vi "Main UI.vi"() -> ()   [LabVIEW 2013]
uses:
  SubVi/Global constant.vi
  <vilib>/regexp/Match Regular Expression.xnode
panel:
  out "Name":string
  out "Info":cluster{"PASS":u32, "Total":u32, "Rate %":dbl}
  out "Test Time (s)":string
  out "MainProcess":T1(ring)
  out "SN":string
  in  "Cancel Button":bool
  out "Model":string
  out "Result":string
  in  "OK Button":bool
  in  "Multicolumn Listbox":i32(listbox)
  out "Horizontal Graduated Bar":u8(slide) max=28 scale=-1.0..8.0
  out "reslut":bool
  out "Boolean":bool
  out "?":string[](array[string])
  out "ItemTag":string
  # "Powered by Domi"
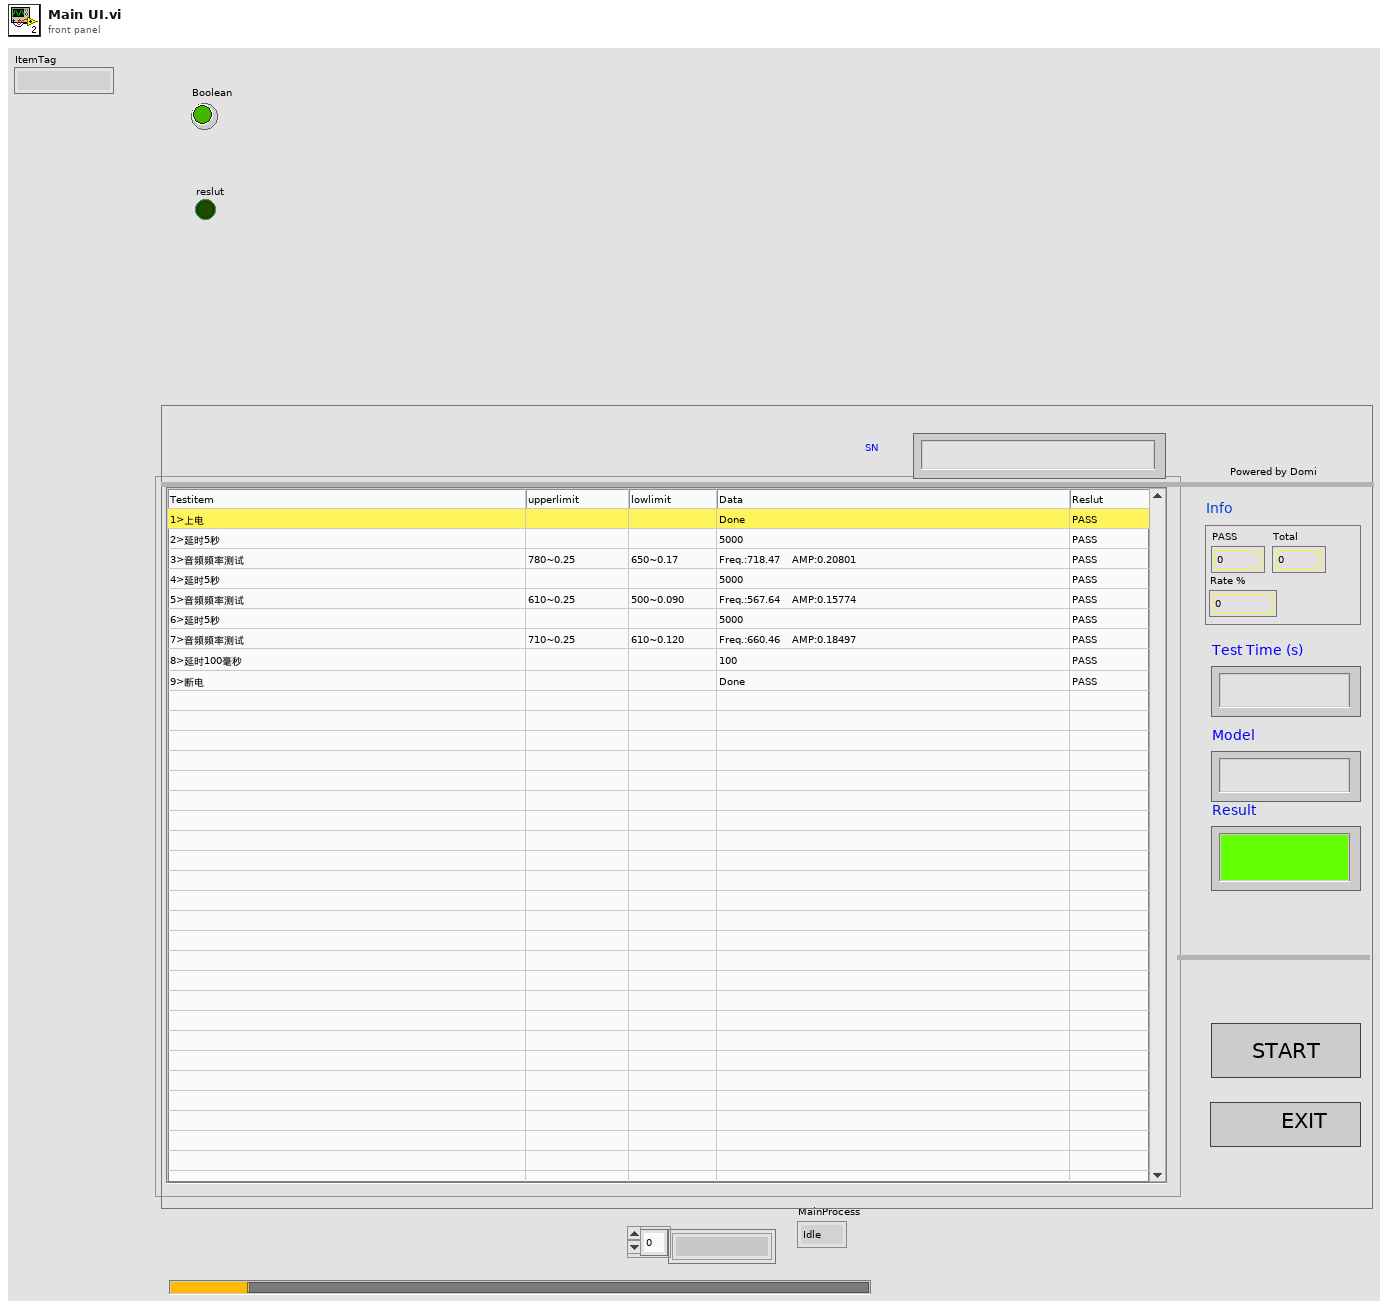
[diagram p1: front panel]
types:
  T1 = enum16{"Idle", "SystemInit", "SpecialEvent", "Barcode(SN)", "TestInitialize", "Test", "TestEnd", "SaveTestData", "Exit", "Stop"}
  T2 = enum8{"Enabled", "Disabled", "Disabled and Grayed Out"}
  T3 = enum16{"open", "replace", "create", "open or create", "replace or create", "replace or create with confirmation"}
  T4 = cluster{"step name 1":string, "updata 2":string, "limitdata 3":string, "load vi name 4":string, "parameter 5":string}
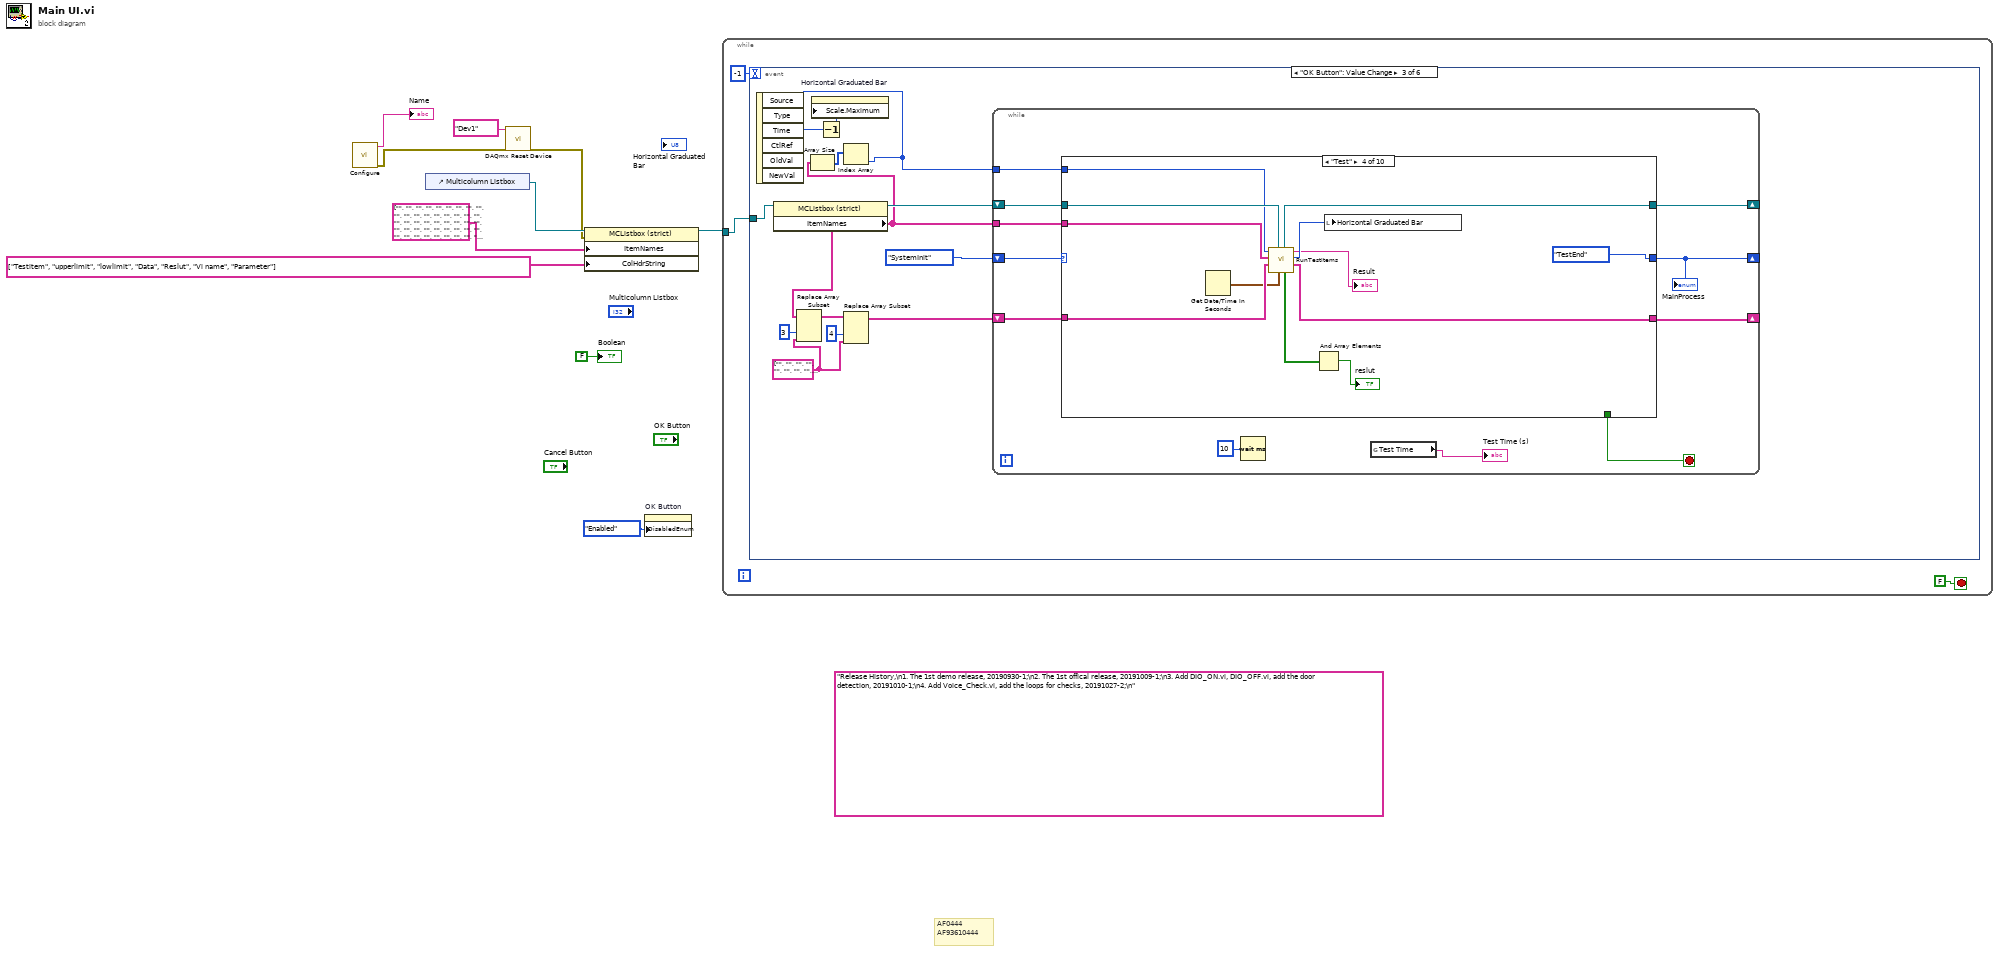
[diagram p0: block diagram]
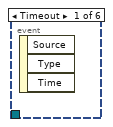
[diagram p2: hidden frame]
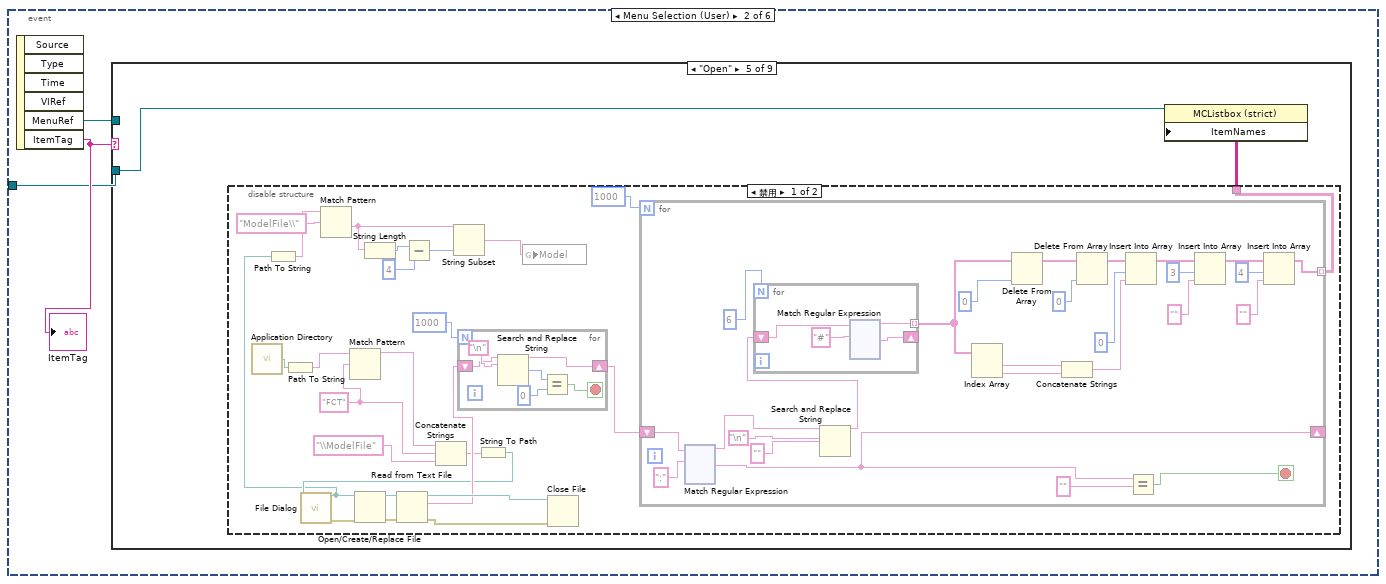
[diagram p3: hidden frame]
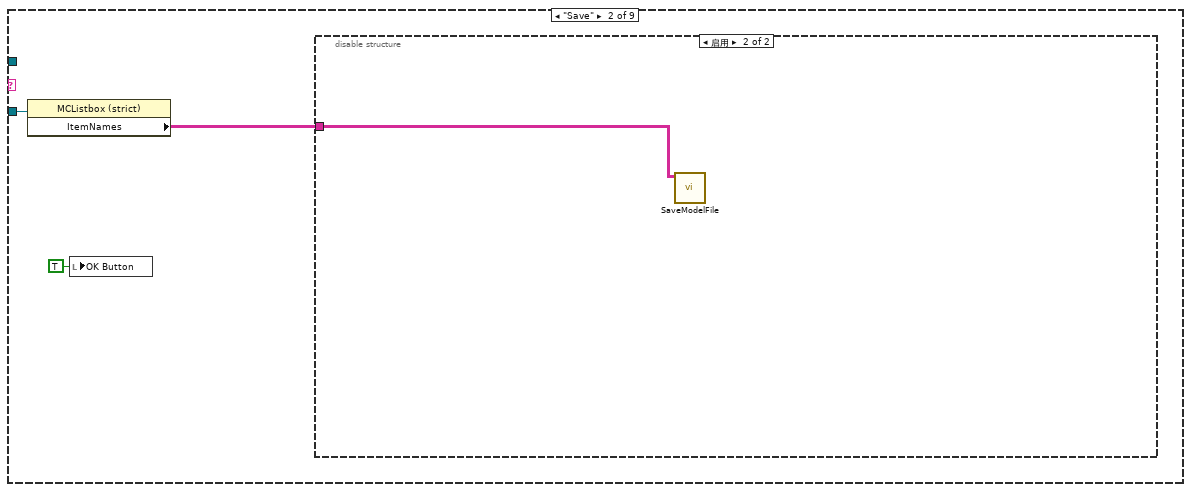
[diagram p5: hidden frame]
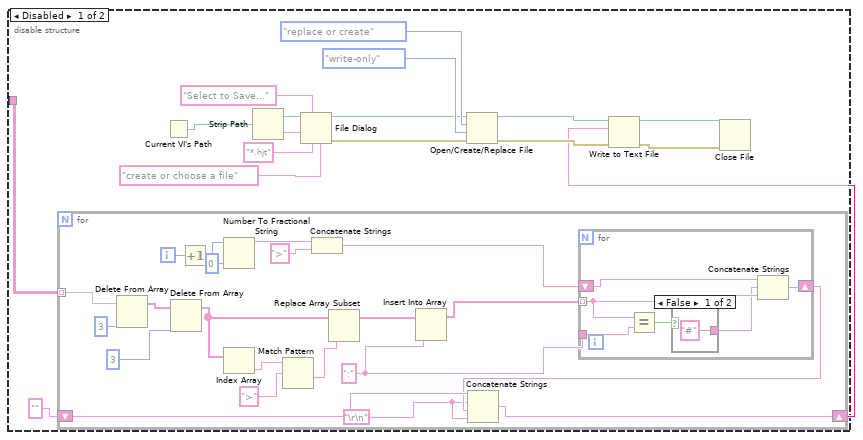
[diagram p6: hidden frame]
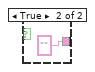
[diagram p7: hidden frame]
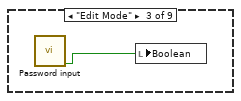
[diagram p8: hidden frame]
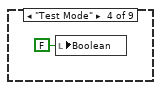
[diagram p9: hidden frame]
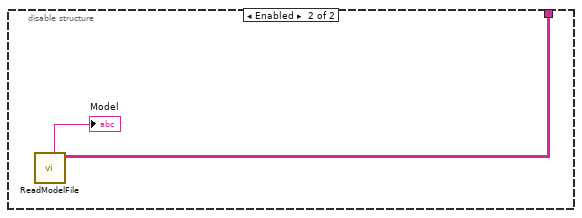
[diagram p10: hidden frame]
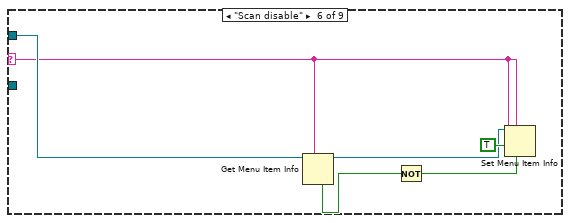
[diagram p11: hidden frame]
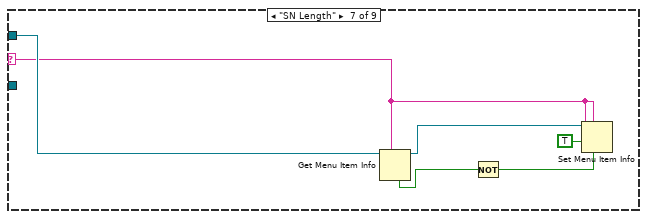
[diagram p12: hidden frame]
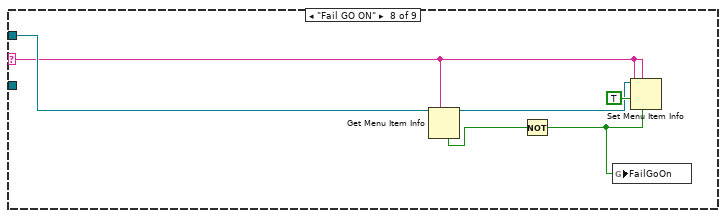
[diagram p13: hidden frame]
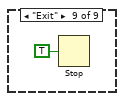
[diagram p14: hidden frame]
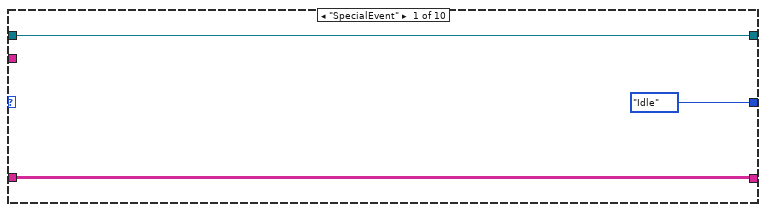
[diagram p15: hidden frame]
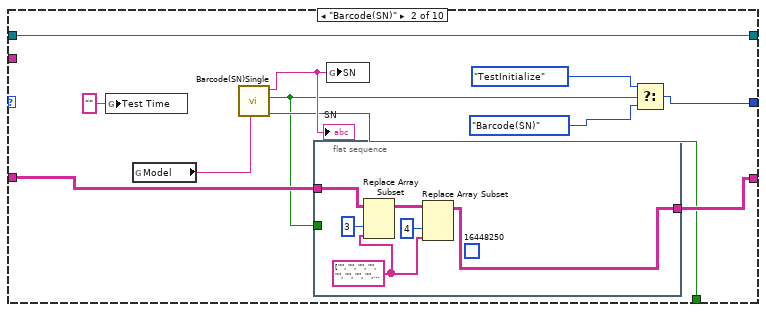
[diagram p16: hidden frame]
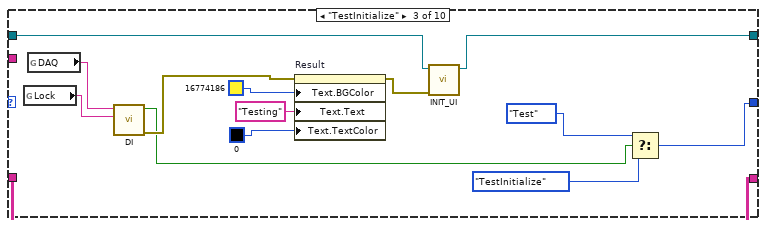
[diagram p17: hidden frame]
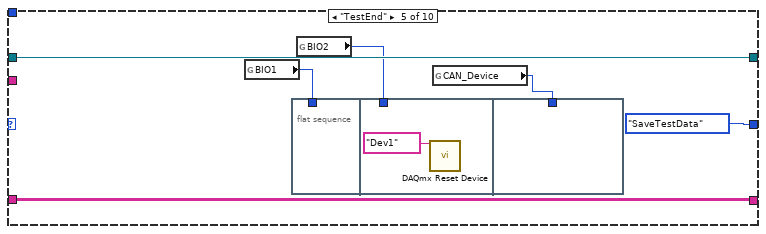
[diagram p18: hidden frame]
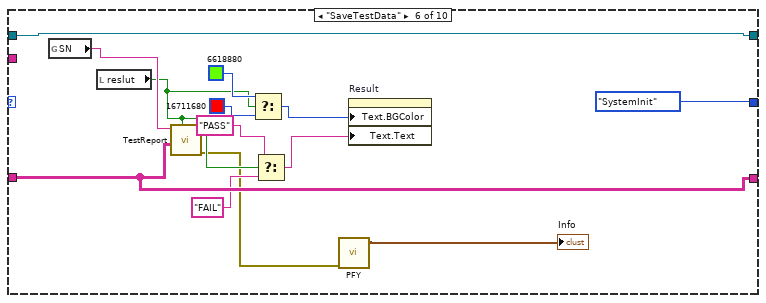
[diagram p19: hidden frame]
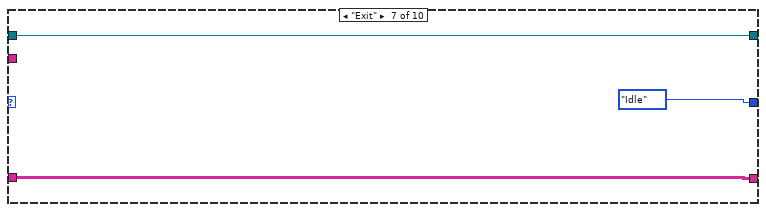
[diagram p20: hidden frame]
diagram:
  (unwired) "Release History,\n1. The 1st demo release, 20190930-1;\n2. The 1st offical release, 20191009-1;\n3. Add DIO_ON.vi, DIO_OFF.vi, add the door detection, 20191010-1;\n4. Add Voice_Check.vi, add the loops for checks, 20191027-2;\n"
  # "AF0444\nAF93610444"
  n1 = call "Configure.vi"() -> ("error out"=w2:errorcluster, "name"=→"Name":string)  [unwired: 10 in]
  n2 = control-ref of="Multicolumn Listbox"() -> (w10:refnum<vi>)
  n3 = call <vilib>:"DAQmx Reset Device.vi"("device in"=tag "Dev1", "error in"=w2) -> ("error out"=w3:errorcluster)  [unwired: 13 in]
  n4 = property class="MCListbox (strict)"(reference=w10, error in=w3, "ItemNames"=string[][] [["", "", "", "", "", "", "", ""], ["", "", "", "", "", "", "", ""], ["", "", "", "", "", "", "", ""], ["", "", "", "", "", "", "", ""], ["", "", "", "", "", "", "", ""], ["", "", "", "", "", "", "", ""], ["", "", "", "", "", "", "", ""], ["", "", "", "", "", "", "", ""], ["", "", "", "", "", "", "", ""], ["", "", "", "", "", "", "", ""], ["", "", "", "", "", "", "", ""], ["", "", "", "", "", "", "", ""], ["", "", "", "", "", "", "", ""], ["", "", "", "", "", "", "", ""], ["", "", "", "", "", "", "", ""], ["", "", "", "", "", "", "", ""], ["", "", "", "", "", "", "", ""], ["", "", "", "", "", "", "", ""], ["", "", "", "", "", "", "", ""], ["", "", "", "", "", "", "", ""], ["", "", "", "", "", "", "", ""], ["", "", "", "", "", "", "", " "], ["", "", "", "", "", "", "", ""], ["", "", "", "", "", "", "", ""], ["", "", "", "", "", "", "", ""], ["", "", "", "", "", "", "", ""], ["", "", "", "", "", "", "", ""], ["", "", "", "", "", "", "", ""], ["", "", "", "", "", "", "", ""], ["", "", "", "", "", "", "", ""], ["", "", "", "", "", "", "", ""], ["", "", "", "", "", "", "", ""], ["", "", "", "", "", "", "", ""], ["", "", "", "", "", "", "", ""], ["", "", "", "", "", "", "", ""], ["", "", "", "", "", "", "", ""], ["", "", "", "", "", "", "", ""], ["", "", "", "", "", "", "", ""], ["", "", "", "", "", "", "", ""], ["", "", "", "", "", "", "", ""], ["", "", "", "", "", "", "", ""], ["", "", "", "", "", "", "", ""]] ("Item Names"), "ColHdrString"=string[] ["Testitem", "upperlimit", "lowlimit", "Data", "Reslut", "Vi name", "Parameter"] ("Row Header Strings[]")) -> (reference out=w7:refnum<vi>)  [unwired: 1 out]
  n5 = property on="OK Button" class="Bool (strict)"("DisabledEnum"=T2."Enabled" ("Disabled")) -> ()  [unwired: 2 in, 2 out]
  n6 = while {
    tunnel: w7 -> [w13]
    stop <- FALSE stop-if-true
    n7 = event shown="[2] \"OK Button\": Value Change" {
      selector: _ -> [_ _ _ _ _ _]
      dyn-events: _ -> [_ _ _ _ _ _]
      timeout: -1 -> [_ _ _ _ _ _]
      tunnel: w13 -> [_ w15 w392 _ w492 w515]
      event Timeout {
        n8 = event-data() -> ()  [unwired: 1 in, 3 out]
      }
      event Menu Selection (User) {
        n9 = event-data() -> ("MenuRef"=w14:refnum<k9>, "ItemTag"=w16:string)  [unwired: 1 in, 4 out]
        "ItemTag" <- w16
        n10 = case shown="\"Open\"" w16 {
          selector: w16 -> [_ _ _ _ _ w362 w368 w377 _]
          tunnel: w15 -> [_ w19 _ _ w70 _ _ _ _]
          tunnel: w14 -> [_ _ _ _ _ w363 w369 w378 _]
          frame "False", Default {
          }
          frame "Save" {
            n11 = property class="MCListbox (strict)"(reference=w19) -> ("ItemNames"=w18:string[][])  [unwired: 1 in, 2 out]
            n12 = local write "OK Button"(TRUE ("OK Button")) -> ()
            n13 = disable-structure shown="启用" {
              disable-tunnel: w18 -> [w26 w66]
              frame Disabled {
                n14 = for {
                  tunnel: w26 -> [w47] mode=indexing
                  shift-right: [w51] -> w23
                  shift-left: "" -> [w50]
                  i -> [w57]
                  w37 = ":" ("new element/subarray")
                  w48 = "\r\n"
                  n15 = Delete From Array(array=w47, index=3) -> (array with subset deleted=w44:string[])  [unwired: 1 in, 1 out]
                  n16 = Delete From Array(array=w44, index=3) -> (array with subset deleted=w42:string[])  [unwired: 1 in, 1 out]
                  n17 = Increment(x=w57) -> (x+1=w56:i32)
                  n18 = Number To Fractional String(number=w56, precision (6)=i16 0) -> (F-format string=w55:string)  [unwired: 2 in]
                  n19 = Index Array(array=w42) -> (element=w43:string)  [unwired: 1 in]
                  n20 = Match Pattern(string=w43, regular expression=">") -> (after substring=w41:string)  [unwired: 1 in, 3 out]
                  n21 = Concatenate Strings(w55, ">") -> (w53:string)
                  n22 = Replace Array Subset(array=w42, new element=w41) -> (w39:string[])  [unwired: 1 in]
                  n23 = Insert Into Array(array=w39, new element=w37) -> (w38:string[])  [unwired: 1 in]
                  n24 = for {
                    shift-right: [w62] -> w49
                    shift-left: w53 -> [w63]
                    tunnel: w38 -> [w60] mode=indexing
                    tunnel: w37 -> [w61]
                    n25 = Equal?(x=w60, y=w61) -> (x = y?=w59:bool)
                    n26 = case shown="False" w59 {
                      tunnel: ["#" ("string") ""] -> w58
                      frame False {
                      }
                      frame True {
                      }
                    }
                    n27 = Concatenate Strings(w63, w58, w60) -> (w62:string)
                  }
                  n28 = Concatenate Strings(w50, w48, w49, w48) -> (w51:string)
                }
                n29 = Current VI's Path() -> (path=w20:path)
                n30 = Strip Path(path=w20) -> (stripped path=w28:path, name=w29:string)
                n31 = File Dialog(4:"create or choose a file" ("pattern label"), 6:"*.hjt" ("pattern (all files)"), 7:"Select to Save..." ("prompt"), 9:w29, 11:w28) -> (0:w31:errorcluster, 3:w30:path)  [unwired: 1 in, 3 out]
                n32 = Open/Create/Replace File(file path (use dialog)=w30, error in=w31, operation (0:open)=T3."replace or create", access (0:read/write)=enum16{"read/write", "read-only", "write-only"}."write-only") -> (refnum out=w24:refnum<file>, error out=w25:errorcluster)  [unwired: 3 out]
                n33 = Write to Text File(file (use dialog)=w24, text=w23, error in=w25) -> (refnum out=w21:refnum<file>, error out=w22:errorcluster)  [unwired: 1 in, 1 out]
                n34 = Close File(refnum=w21, error in=w22) -> ()  [unwired: 2 out]
              }
              frame Enabled {
                n35 = call "SaveModelFile.vi"("ItemNames"=w66) -> ()  [unwired: 10 in, 1 out]
              }
            }
          }
          frame "Edit Mode" {
            n36 = call "Password input.vi"() -> ("Boolean"=w67:bool)  [unwired: 10 in, 1 out]
            n37 = local write "Boolean"(w67) -> ()
          }
          frame "Test Mode" {
            n38 = local write "Boolean"(FALSE ("Boolean")) -> ()
          }
          frame "Open" {
            n39 = disable-structure shown="禁用" {
              disable-tunnel: [w91 w361] -> w69
              frame Disabled {
                w75 = "FCT" ("search string")
                n40 = call <vilib>:"Application Directory.vi"() -> ("Application Directory"=w78:path)
                n41 = Path To String(path=w78) -> (string=w77:string)
                n42 = Match Pattern(string=w77, regular expression=w75) -> (before substring=w76:string)  [unwired: 1 in, 3 out]
                n43 = Concatenate Strings(w76, w75, "\\ModelFile" ("string")) -> (w73:string)
                n44 = String To Path(string=w73) -> (path=w72:path)
                n45 = call "File Dialog"("start path"=w72) -> ("selected path"=w71:path, "error out"=w93:errorcluster)  [unwired: 11 in, 2 out]
                n46 = Path To String(path=w71) -> (string=w88:string)
                n47 = Match Pattern(string=w88, regular expression="ModelFile\\") -> (after substring=w83:string)  [unwired: 1 in, 3 out]
                n48 = Open/Create/Replace File(file path (use dialog)=w71, error in=w93) -> (refnum out=w94:refnum<file>, error out=w95:errorcluster)  [unwired: 4 in, 1 out]
                n49 = String Length(string=w83) -> (length=w86:i32)
                n50 = Read from Text File(file (use dialog)=w94, error in=w95) -> (refnum out=w89:refnum<file>, text=w81:string, error out=w90:errorcluster)  [unwired: 2 in, 1 out]
                n51 = Subtract(x=w86, y=4) -> (x-y=w84:i32)
                n52 = String Subset(string=w83, length (rest)=w84) -> (substring=w79:string)  [unwired: 1 in]
                n53 = for {
                  N: 1000 -> [_]
                  shift-right: [w99] -> w80
                  shift-left: w81 -> [w100]
                  stop <- w96 stop-if-true
                  n54 = Search and Replace String(input string=w100, search string="\n") -> (result string=w99:string, number of replacements=w98:i32)  [unwired: 6 in, 2 out]
                  n55 = Equal?(x=w98, y=0) -> (x = y?=w96:bool)
                }
                n56 = global write "Global constant.vi" "Model"(w79) -> ()
                n57 = Close File(refnum=w89, error in=w90) -> ()  [unwired: 2 out]
                n58 = for {
                  N: 1000 -> [_]
                  shift-right: [w108] -> _
                  shift-left: w80 -> [w127]
                  tunnel: [w109] -> w91 mode=indexing
                  stop <- w106 stop-if-true
                  n59 = xnode ("Match Regular Expression")("input string"=w127, "regular expression"=":") -> ("before match"=w105:string, "after match"=w108:string)  [unwired: 4 in, 3 out]
                  n60 = Search and Replace String(input string=w105, search string="\n" ("Line Feed Constant"), replace string="" ("replace string (\"\")")) -> (result string=w102:string)  [unwired: 5 in, 3 out]
                  n61 = for {
                    N: 6 -> [_]
                    shift-right: [w129] -> _
                    shift-left: w102 -> [w130]
                    tunnel: [w128] -> w122 mode=indexing
                    n62 = xnode "Match Regular Expression"("input string"=w130, "regular expression"="#") -> ("before match"=w128:string, "after match"=w129:string)  [unwired: 4 in, 3 out]
                  }
                  n63 = Index Array(array=w122) -> (element #1=w123:string, element #2=w124:string)  [unwired: 2 in]
                  n64 = Delete From Array(array=w122, index=0) -> (array with subset deleted=w121:string[])  [unwired: 1 in, 1 out]
                  n65 = Concatenate Strings(w123, w124) -> (w117:string)
                  n66 = Delete From Array(array=w121, index=0) -> (array with subset deleted=w118:string[])  [unwired: 1 in, 1 out]
                  n67 = Insert Into Array(array=w118, index=0, new element=w117) -> (w115:string[])
                  n68 = Equal?(x=w108, y="") -> (x = y?=w106:bool)
                  n69 = Insert Into Array(array=w115, index=3, new element="" ("new element/subarray")) -> (w112:string[])
                  n70 = Insert Into Array(array=w112, index=4, new element="" ("new element/subarray")) -> (w109:string[])
                }
              }
              frame Enabled {
                n71 = call "ReadModelFile.vi"() -> ("out"=w361:string[][], "Model"=→"Model":string)  [unwired: 9 in, 1 out]
              }
            }
            n72 = property class="MCListbox (strict)"(reference=w70, "ItemNames"=w69) -> ()  [unwired: 1 in, 2 out]
          }
          frame "Scan disable" {
            n73 = Get Menu Item Info(7:w362, 11:w363) -> (3:w364:refnum<k9>, 4:w366:bool)  [unwired: 1 in, 5 out]
            n74 = Not(x=w366) -> (.not. x?=w365:bool)
            n75 = Set Menu Item Info(6:w365, 7:w362, 9:TRUE ("enabled"), 10:w362, 11:w364) -> ()  [unwired: 2 in, 2 out]
          }
          frame "SN Length" {
            n76 = Get Menu Item Info(7:w368, 11:w369) -> (3:w370:refnum<k9>, 4:w372:bool)  [unwired: 1 in, 5 out]
            n77 = Not(x=w372) -> (.not. x?=w371:bool)
            n78 = Set Menu Item Info(6:w371, 7:w368, 9:TRUE ("enabled"), 10:w368, 11:w370) -> ()  [unwired: 2 in, 2 out]
          }
          frame "Fail GO ON" {
            n79 = Get Menu Item Info(7:w377, 11:w378) -> (3:w375:refnum<k9>, 4:w376:bool)  [unwired: 1 in, 5 out]
            n80 = Not(x=w376) -> (.not. x?=w374:bool)
            n81 = global write "Global constant.vi" "FailGoOn"(w374) -> ()
            n82 = Set Menu Item Info(6:w374, 7:w377, 9:TRUE ("enabled"), 10:w377, 11:w375) -> ()  [unwired: 2 in, 2 out]
          }
          frame "Exit" {
            n83 = Stop(stop? (T)=TRUE) -> ()
          }
        }
      }
      event "OK Button": Value Change {
        w390 = string[] ["", "", "", "", "", "", "", "", "", "", "", "", "", "", "", "", "", "", "", "", "", "", "", "", "", "", "", "", "", "", "", "", "", "", "", "", "", "", "", "", "", "", "", "", "", "", "", "", "", "", "", "", "", "", "", "", "", "", "", "", "", "", "", "", "", "", "", "", "", "", "", "", "", "", "", "", "", "", "", "", "", "", "", "", "", "", "", "", "", "", "", "", "", "", "", "", "", "", "", "", ""] ("new element/subarray")
        n84 = event-data() -> ()  [unwired: 1 in, 6 out]
        n85 = property class="MCListbox (strict)"(reference=w392) -> (reference out=w384:refnum<vi>, "ItemNames"=w381:string[][])  [unwired: 1 in, 1 out]
        n86 = Replace Array Subset(array=w381, new element=w390, index (col)=3 ("disabled index (col)")) -> (w389:string[][])  [unwired: 1 in]
        n87 = Array Size(array=w381) -> (size(s)=w387:i32[])
        n88 = Index Array(array=w387) -> (element=w383:i32)  [unwired: 1 in]
        n89 = Decrement(x=w383) -> (x-1=w386:i32)
        n90 = property on="Horizontal Graduated Bar" class="Slide (strict)"("Scale.Maximum"=w386) -> ()  [unwired: 2 in, 2 out]
        n91 = Replace Array Subset(array=w389, new element=w390, index (col)=4 ("disabled index (col)")) -> (w382:string[][])  [unwired: 1 in]
        n92 = while {
          shift-right: [w399] -> _
          shift-left: T1."SystemInit" ("MainProcess") -> [w403]
          tunnel: w383 -> [w398]
          tunnel: w381 -> [w396]
          shift-right: [w395] -> _
          shift-left: w382 -> [w397]
          shift-right: [w394] -> _
          shift-left: w384 -> [w400]
          stop <- w402 stop-if-true
          n93 = case shown="\"Test\"" w403 {
            tunnel: [_ w410 _ _ _ _ _ TRUE _ _] -> w402
            tunnel: w400 -> [w404 w408 w433 w449 w453 w467 w470 w473 w481 w487]
            tunnel: [T1."Idle" ("MainProcess") w414 w425 T1."TestEnd" ("MainProcess") T1."SaveTestData" ("MainProcess") T1."SystemInit" ("MainProcess") T1."Idle" ("MainProcess") T1."SystemInit" ("MainProcess") T1."Barcode(SN)" ("MainProcess") T1."SystemInit" ("MainProcess")] -> w399
            tunnel: w398 -> [_ _ _ w448 _ _ _ _ _ _]
            tunnel: w397 -> [w406 w412 w437 w447 w455 w466 w471 w475 w479 w489]
            tunnel: w396 -> [_ _ _ w446 _ _ _ _ _ _]
            tunnel: [w406 w411 w437 w441 w455 w466 w471 w475 w479 w489] -> w395
            tunnel: [w404 w408 w432 w439 w453 w467 w470 w473 w478 w487] -> w394
            frame "SpecialEvent" {
            }
            frame "Barcode(SN)" {
              n94 = global write "Global constant.vi" "Test Time"("" ("Test Time")) -> ()
              n95 = global read "Global constant.vi" "Model"() -> (w417:string)
              n96 = call "Barcode(SN)Single.vi"("Model"=w417) -> ("Stop"=w410:bool, "SNCheck"=w409:bool, "Barcode out:"=w413:string)  [unwired: 7 in, 1 out]
              "SN" <- w413
              n97 = flat-sequence {
                tunnel: w412 -> [w418]
                tunnel: [w419] -> w411
                tunnel: w409 -> [_]
                frame #0 {
                  (unwired) u32 16448250
                  w422 = string[] ["", "", "", "", "", "", "", "", "", "", "", "", "", "", "", "", "", "", "", "", "", "", "", "", "", "", "", "", "", "", "", "", "", "", "", "", "", "", "", "", "", "", "", "", "", "", "", "", "", "", "", "", "", "", "", "", "", "", "", "", "", "", "", "", "", "", "", "", "", "", "", "", "", "", "", "", "", "", "", "", "", "", "", "", "", "", "", "", "", "", "", "", "", "", "", "", "", "", "", "", ""] ("new element/subarray")
                  n98 = Replace Array Subset(array=w418, new element=w422, index (col)=3 ("disabled index (col)")) -> (w421:string[][])  [unwired: 1 in]
                  n99 = Replace Array Subset(array=w421, new element=w422, index (col)=4 ("disabled index (col)")) -> (w419:string[][])  [unwired: 1 in]
                }
              }
              n100 = global write "Global constant.vi" "SN"(w413) -> ()
              n101 = Select(t=T1."TestInitialize" ("MainProcess"), s=w409, f=T1."Barcode(SN)" ("MainProcess")) -> (s? t:f=w414:T1)
            }
            frame "TestInitialize" {
              n102 = global read "Global constant.vi" "Lock"() -> (w428:string)
              n103 = global read "Global constant.vi" "DAQ"() -> (w429:tag)
              n104 = call "DI.vi"("Line"=w428, "Device"=w429) -> ("error out"=w430:errorcluster, "data"=w427:bool)  [unwired: 8 in]
              n105 = property on="Result" class="Str"(error in=w430, "Text.BGColor"=u32 16774186, "Text.Text"="Testing", "Text.TextColor"=u32 0) -> (error out=w431:errorcluster)  [unwired: 1 in, 1 out]
              n106 = call "INIT_UI.vi"("error in (no error)"=w431, "reference"=w433) -> ("reference out"=w432:refnum<vi>)  [unwired: 8 in, 1 out]
              n107 = Select(t=T1."Test" ("MainProcess"), s=w427, f=T1."TestInitialize" ("MainProcess")) -> (s? t:f=w425:T1)
            }
            frame "Test" {
              n108 = Get Date/Time In Seconds() -> (seconds since 1Jan1904=w438:timestamp)
              n109 = call "RunTestItems.vi"("seconds since 1Jan1904"=w438, "Multicolumn Listbox"=w449, "Item in"=w447, "ItemNames"=w446, "steps"=w448) -> ("Items out"=w441:string[][], "Horizontal Graduated Bar"=w443:u8, 3:"Result"=→"Result":string, 4:"Result"=w444:bool[], "Multicolumn Listbox 2"=w439:refnum<vi>)  [unwired: 1 in, 1 out]
              n110 = And Array Elements(Boolean array=w444) -> (logical AND=→"reslut":bool)
              n111 = local write "Horizontal Graduated Bar"(w443) -> ()
            }
            frame "TestEnd" {
              n112 = global read "Global constant.vi" "BIO1"() -> (w452:i32)
              n113 = flat-sequence {
                tunnel: w452 -> [_]
                tunnel: w451 -> [_]
                tunnel: w450 -> [_]
                frame #0 {
                }
                frame #1 {
                  n114 = call <vilib>:"DAQmx Reset Device.vi"("device in"=tag "Dev1") -> ()  [unwired: 14 in, 1 out]
                }
                frame #2 {
                }
              }
              n115 = global read "Global constant.vi" "BIO2"() -> (w451:i32)
              n116 = global read "Global constant.vi" "CAN_Device"() -> (w450:i32)
            }
            frame "SaveTestData" {
              n117 = global read "Global constant.vi" "SN"() -> (w468:string)
              n118 = local read "reslut"() -> (w462:bool)
              n119 = call "TestReport.vi"("reslut"=w462, "Items out"=w466, "SN"=w468) -> ("error out"=w458:errorcluster)  [unwired: 8 in]
              n120 = Select(t=u32 6618880, s=w462, f=u32 16711680) -> (s? t:f=w464:u32)
              n121 = Select(t="PASS", s=w462, f="FAIL") -> (s? t:f=w459:string)
              n122 = call "PFY.vi"("错误输入"=w458) -> ("输出簇"=→"Info":cluster{"PASS":u32, "Total":u32, "Rate":dbl})  [unwired: 9 in, 1 out]
              n123 = property on="Result" class="Str"("Text.BGColor"=w464, "Text.Text"=w459) -> ()  [unwired: 2 in, 2 out]
            }
            frame "Exit" {
            }
            frame "Stop" {
            }
            frame "SystemInit" {
              n124 = First Call?() -> (First Call?: T/F=w477:bool)
              n125 = case shown="True" w477 {
                frame False {
                }
                frame True {
                  n126 = call "Configure.vi"() -> ("error out"=w486:errorcluster)  [unwired: 10 in, 1 out]
                  n127 = call "PFY.vi"("错误输入"=w486) -> ("输出簇"=w485:cluster{"PASS":u32, "Total":u32, "Rate":dbl})  [unwired: 9 in, 1 out]
                  n128 = local write "Info"(w485) -> ()
                }
              }
              n129 = case shown="True" w477 {
                tunnel: w481 -> [w482 w484]
                tunnel: [w482 w483] -> w478
                frame False {
                }
                frame True {
                  n130 = call "INIT_UI.vi"("reference"=w484) -> ("reference out"=w483:refnum<vi>)  [unwired: 9 in, 1 out]
                }
              }
            }
            frame "Idle" {
            }
          }
          "MainProcess" <- w399
          n131 = Wait (ms)(milliseconds to wait=u32 10) -> ()  [unwired: 1 out]
          n132 = global read "Global constant.vi" "Test Time"() -> (→"Test Time (s)":string)
        }
      }
      event "Cancel Button": Value Change {
        n133 = event-data() -> ()  [unwired: 1 in, 6 out]
        n134 = flat-sequence {
          frame #0 {
            # "CLOSE ALL"
          }
          frame #1 {
            n135 = control-ref of="This VI"() -> (w490:refnum<vi>)
            n136 = invoke class="VI" method="FP.Close"(reference=w490) -> ()  [unwired: 2 in, 3 out]
          }
        }
      }
      event "Multicolumn Listbox": Double Click {
        n137 = event-data() -> ()  [unwired: 1 in, 9 out]
        n138 = local read "Boolean"() -> (w491:bool)
        n139 = case shown="True" w491 {
          tunnel: w492 -> [_ w513]
          frame False {
          }
          frame True {
            n140 = property class="MCListbox (strict)"(reference=w513) -> (reference out=w506:refnum<vi>, "ItemNames"=w503:string[][], "Value"=w504:i32)  [unwired: 1 in, 1 out]
            n141 = Index Array(array=w503, index (row)=w504) -> (element=w512:string[])  [unwired: 1 in]
            n142 = Index Array(array=w512) -> (element #1=w510:string, element #2=w509:string, element #3=w508:string, element #6=w507:string, element #7=w493:string)  [unwired: 7 in, 2 out]
            n143 = Bundle By Name(cluster=T4 {"step name 1"="", "updata 2"="", "limitdata 3"="", "load vi name 4"="", "parameter 5"=""} ("IN"), "step name 1"=w510, "updata 2"=w509, "limitdata 3"=w508, "load vi name 4"=w507, "parameter 5"=w493) -> (w501:T4)
            n144 = call "Parameter Setting.vi"("TEST INFO"=w501) -> ("IN 2"=w502:T4)  [unwired: 10 in]
            n145 = Cluster To Array(cluster=w502) -> (array=w500:string[])
            n146 = Insert Into Array(array=w500, index=3, new element="" ("new element/subarray")) -> (w498:string[])
            n147 = Insert Into Array(array=w498, index=4, new element="" ("new element/subarray")) -> (w494:string[])
            n148 = Replace Array Subset(array=w503, new element=w494, index (row)=w504) -> (w505:string[][])  [unwired: 1 in]
            n149 = property class="MCListbox (strict)"(reference=w506, "ItemNames"=w505) -> ()  [unwired: 1 in, 2 out]
          }
        }
      }
      event "Multicolumn Listbox": Shortcut Menu Selection (User) {
        n150 = event-data() -> ("ItemTag"=w516:string)  [unwired: 1 in, 7 out]
        n151 = local read "Boolean"() -> (w514:bool)
        n152 = case shown="True" w514 {
          tunnel: w516 -> [_ w518]
          tunnel: w515 -> [_ w517]
          frame False {
          }
          frame True {
            n153 = case shown="\"COM\"" w518 {
              tunnel: w517 -> [w524 w525 w531 w540 w544 w551]
              frame "A", Default {
                n154 = property class="MCListbox (strict)"(reference=w524) -> (reference out=w523:refnum<vi>, "Value"=w522:i32, "ItemNames"=w519:string[][])  [unwired: 1 in, 1 out]
                n155 = Insert Into Array(array=w519, index (row)=w522, new element=string[] ["A45", "A", "A4", "66AAA", "AA"] ("new element/subarray")) -> (w520:string[][])  [unwired: 1 in]
                n156 = property class="MCListbox (strict)"(reference=w523, "ItemNames"=w520) -> ()  [unwired: 1 in, 2 out]
              }
              frame "B" {
                n157 = property class="MCListbox (strict)"(reference=w525) -> (reference out=w530:refnum<vi>, "Value"=w529:i32, "ItemNames"=w526:string[][])  [unwired: 1 in, 1 out]
                n158 = Insert Into Array(array=w526, index (row)=w529, new element=string[] ["B45", "B", "B4", "BBBBB6AAA", "BBBBBBA"] ("new element/subarray")) -> (w527:string[][])  [unwired: 1 in]
                n159 = property class="MCListbox (strict)"(reference=w530, "ItemNames"=w527) -> ()  [unwired: 1 in, 2 out]
              }
              frame "COM" {
                n160 = property class="MCListbox (strict)"(reference=w531) -> (reference out=w536:refnum<vi>, "Value"=w535:i32, "ItemNames"=w532:string[][])  [unwired: 1 in, 1 out]
                n161 = Insert Into Array(array=w532, index (row)=w535, new element=string[] ["COM1", "H", "L", "", ""] ("new element/subarray")) -> (w533:string[][])  [unwired: 1 in]
                n162 = property class="MCListbox (strict)"(reference=w536, "ItemNames"=w533) -> ()  [unwired: 1 in, 2 out]
              }
              frame "Paste" {
                n163 = property class="MCListbox (strict)"(reference=w540) -> (reference out=w538:refnum<vi>, "Value"=w541:i32, "ItemNames"=w542:string[][])  [unwired: 1 in, 1 out]
                n164 = local read item#2() -> (w539:string[])
                n165 = Replace Array Subset(array=w542, new element=w539, index (row)=w541) -> (w537:string[][])  [unwired: 1 in]
                n166 = property class="MCListbox (strict)"(reference=w538, "ItemNames"=w537) -> ()  [unwired: 1 in, 2 out]
              }
              frame "Delete" {
                n167 = property class="MCListbox (strict)"(reference=w544) -> (reference out=w547:refnum<vi>, "Value"=w543:i32, "ItemNames"=w545:string[][])  [unwired: 1 in, 1 out]
                n168 = Delete From Array(array=w545, index (row)=w543) -> (array with subset deleted=w546:string[][])  [unwired: 2 in, 1 out]
                n169 = property class="MCListbox (strict)"(reference=w547, "ItemNames"=w546) -> ()  [unwired: 1 in, 2 out]
              }
              frame "Copy" {
                n170 = property class="MCListbox (strict)"(reference=w551) -> ("Value"=w549:i32, "ItemNames"=w550:string[][])  [unwired: 1 in, 2 out]
                n171 = Index Array(array=w550, index (row)=w549) -> (element=→"?":string[])  [unwired: 1 in]
              }
            }
          }
        }
      }
    }
  }
  "Boolean" <- FALSE ("Boolean")
